vi "Annotating a Picture.vi"() -> ()   [LabVIEW 2023]
doc: "This example demonstrates how to add annotations, or additional images, to a starting image in a <b>2D Picture</b> indicator. The example keeps track of the parts of the image that have been annotated so that the annotations can also be removed if necessary. Finally, the example includes a button to save the modified image (including annotations) to a new image file."
uses:
  <vilib>/Utility/miscctls.llb/LVPoint32TypeDef.ctl
panel:
  in  "Save Image":bool
  in  "Stop":bool
  in  "Load Image":bool
  out "Image":picture
  # "Overview: Demonstrates how to add images as annotations to an existing image displayed in a 2D Picture indicator.\nInstructions: \n1. Run the VI.\n2. Click Load Image to load a JPG file into the picture indicator (this example loads the 'sample_board.jpg' image file).\n3. Right-click in the picture and select one of the Draw Annotation options. Observe the annotation that is added to the image.\n4. Right-click any annotation you have created and select Remove Annotation to see it be removed from the image.\n5. Click Save Image to save the image to a new JPG file. The new JPG file will contain the original image, along with any annotations that were created.\n6. Click Stop to stop the VI."
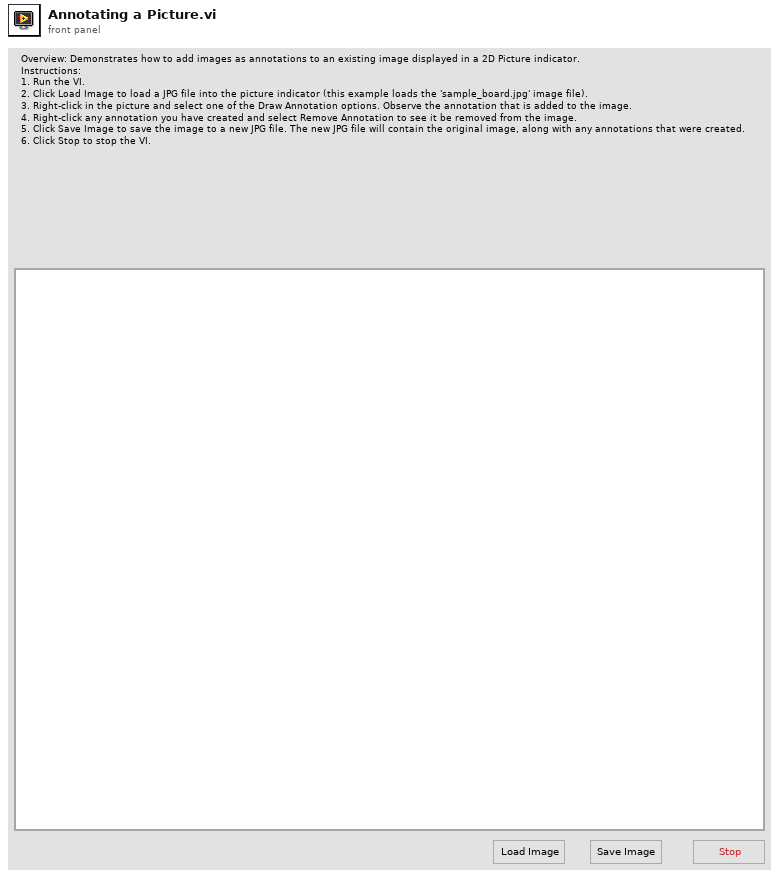
[diagram p1: front panel]
types:
  T1 = cluster{"left":i16, "top":i16, "right":i16, "bottom":i16}[]
  T2 = typedef "LVPoint32TypeDef.ctl" = cluster{"Horizontal":i32, "Vertical":i32}
  T3 = typedef "imagedata.ctl" = cluster{"image type":i32, "image depth":i32, "image":u8[], "mask":u8[], "colors":u32[], "Rectangle":cluster{"left":i16, "top":i16, "right":i16, "bottom":i16}}
  T4 = cluster{"left":i16, "top":i16, "right":i16, "bottom":i16}
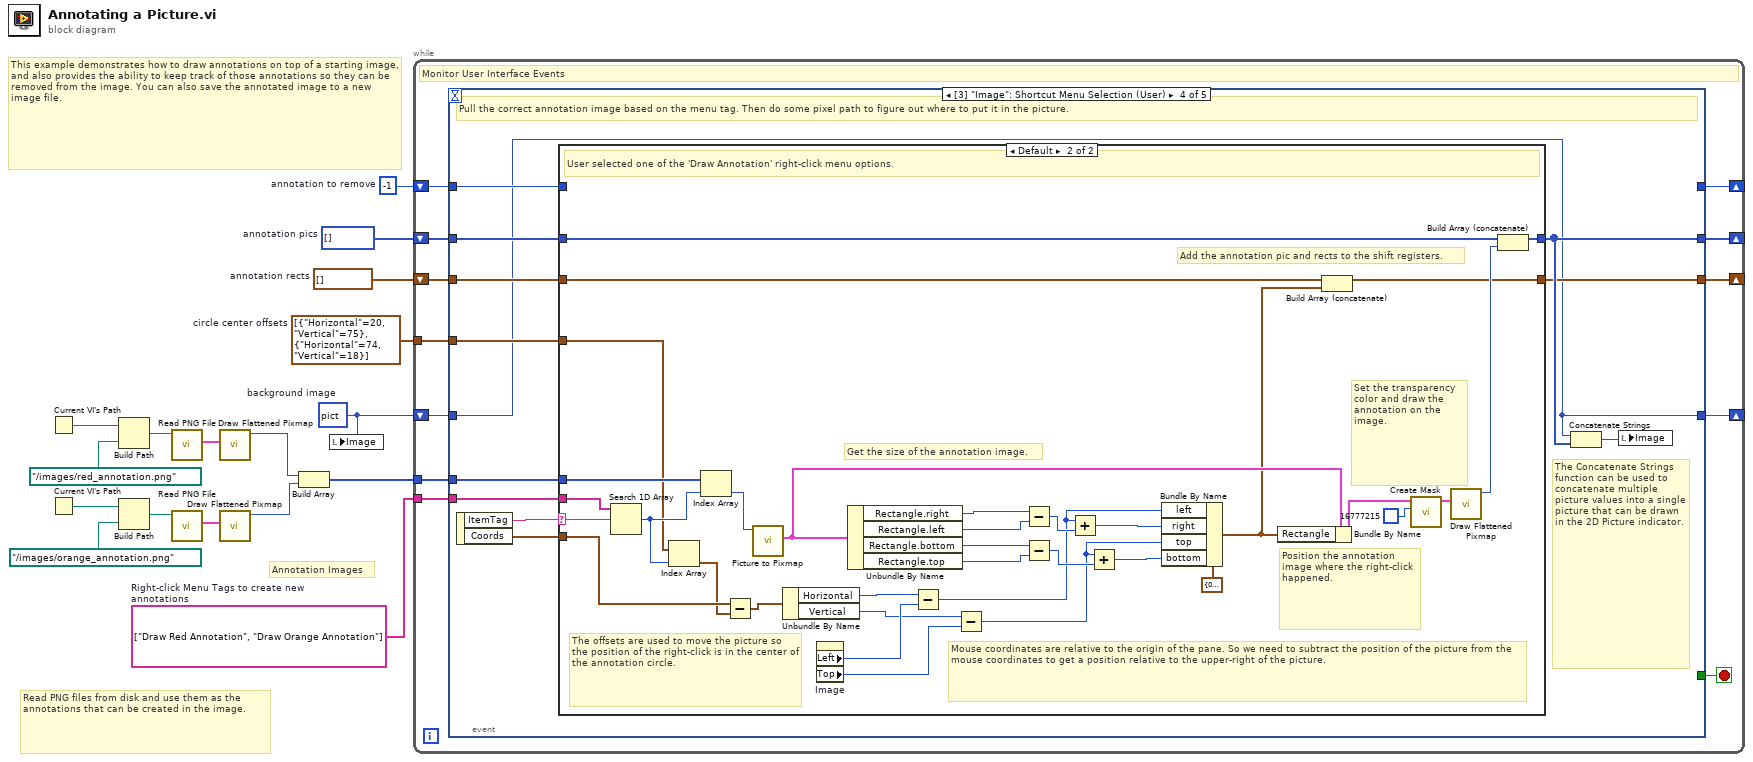
[diagram p0: block diagram]
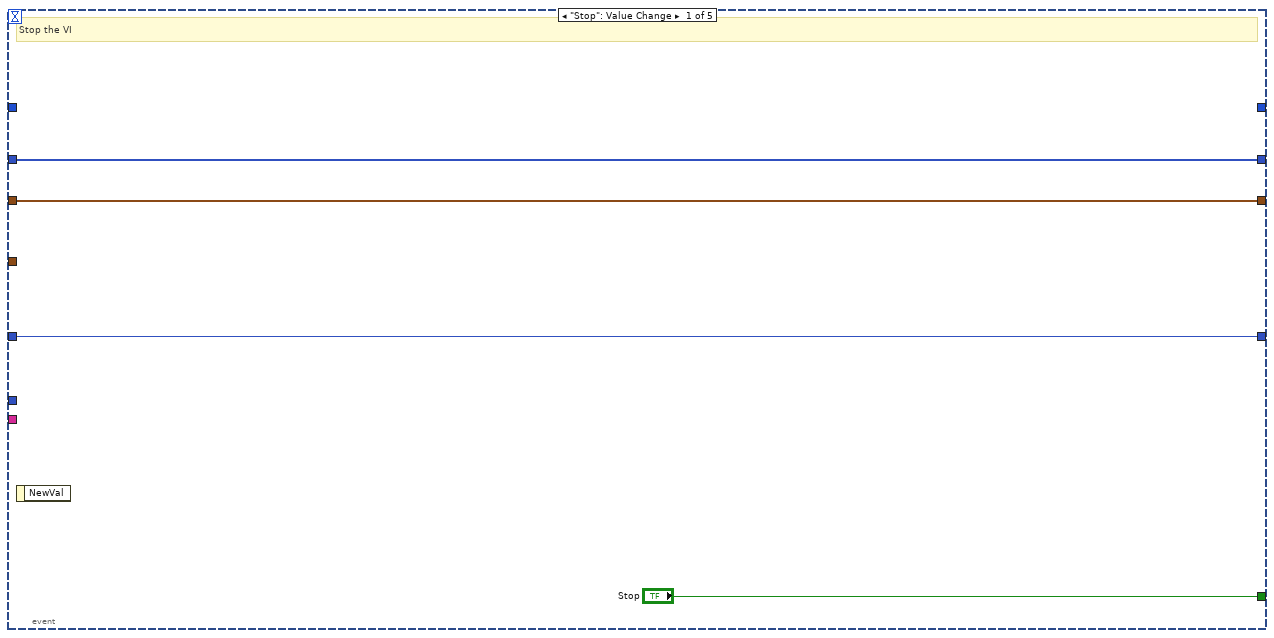
[diagram p2: hidden frame]
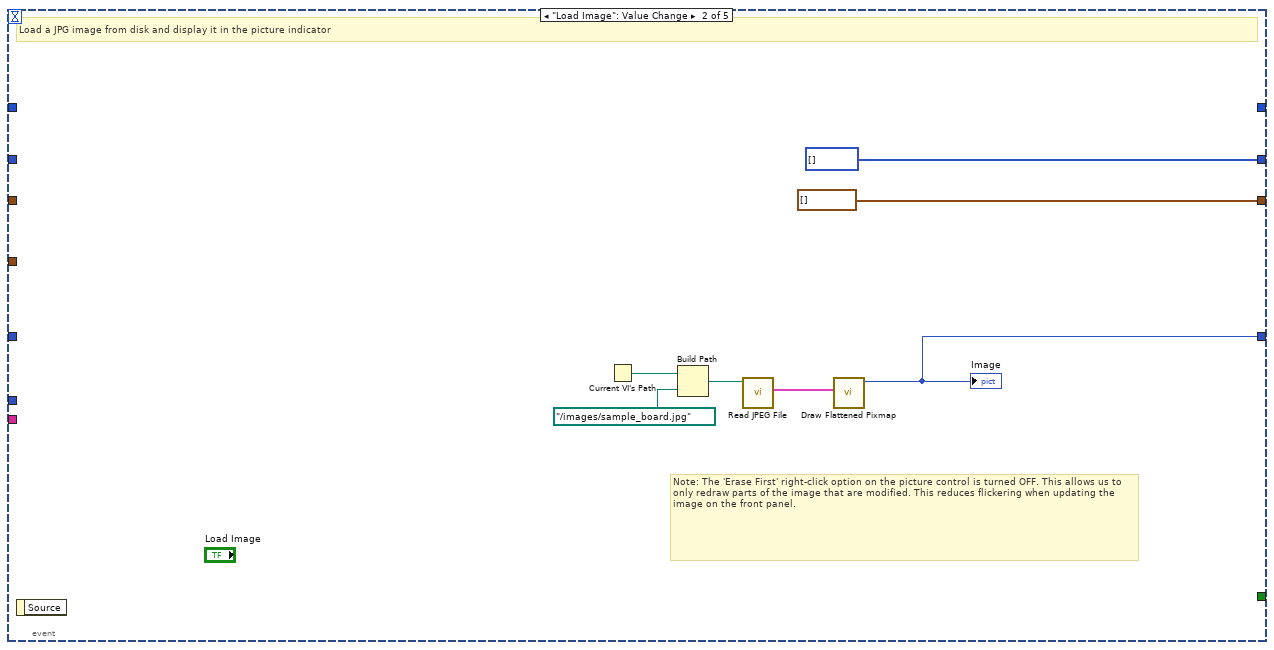
[diagram p3: hidden frame]
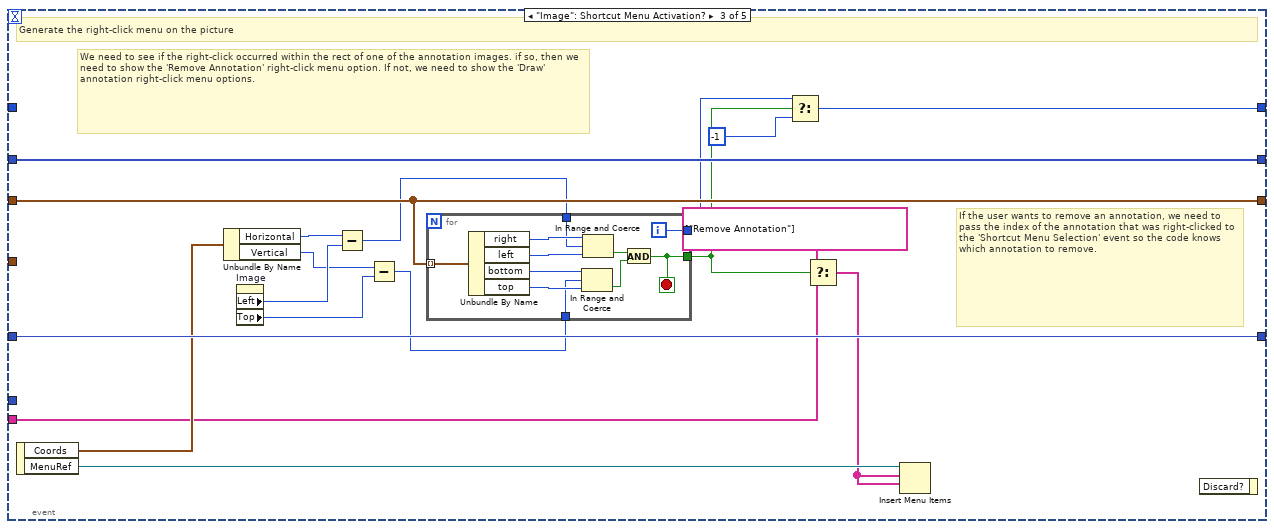
[diagram p4: hidden frame]
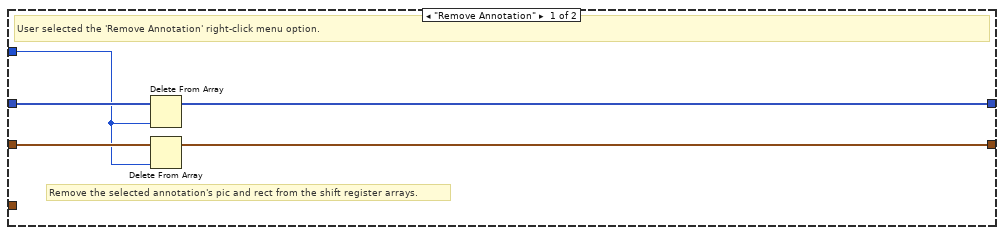
[diagram p5: hidden frame]
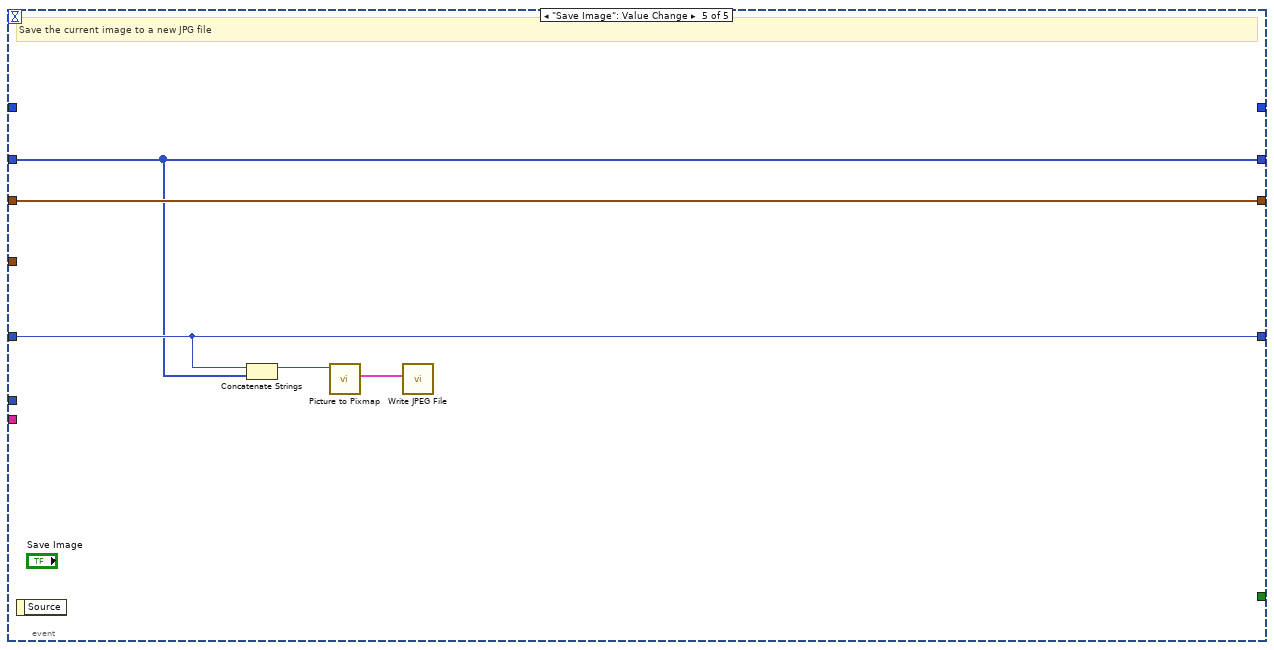
[diagram p6: hidden frame]
diagram:
  w9 = -1  # annotation to remove
  w10 = picture[] []  # annotation pics
  w11 = T1 []  # annotation rects
  w12 = T2[] [{"Horizontal"=20, "Vertical"=75}, {"Horizontal"=74, "Vertical"=18}]  # circle center offsets
  w15 = picture data[5B]  # background image
  w17 = string[] ["Draw Red Annotation", "Draw Orange Annotation"]  # Right-click Menu Tags to create new annotations
  # "This example demonstrates how to draw annotations on top of a starting image, and also provides the ability to keep track of those annotations so they can be removed from the image. You can also save the annotated image to a new image file."
  # "Annotation Images"
  # "Read PNG files from disk and use them as the annotations that can be created in the image."
  n1 = Current VI's Path() -> (path=w8:path)
  n2 = Current VI's Path() -> (path=w1:path)
  n3 = Build Path(base path=w8, name or relative path=path "../images/red_annotation.png") -> (appended path=w7:path)
  n4 = Build Path(base path=w1, name or relative path=path "../images/orange_annotation.png") -> (appended path=w2:path)
  n5 = call <vilib>:"Read PNG File.vi"("path to PNG file"=w7) -> ("image data"=w5:T3)  [unwired: 8 in, 2 out]
  n6 = call <vilib>:"Read PNG File.vi"("path to PNG file"=w2) -> ("image data"=w4:T3)  [unwired: 8 in, 2 out]
  n7 = call <vilib>:"Draw Flattened Pixmap.vi"("image data"=w5) -> ("new picture"=w14:picture)  [unwired: 8 in]
  n8 = call <vilib>:"Draw Flattened Pixmap.vi"("image data"=w4) -> ("new picture"=w13:picture)  [unwired: 8 in]
  n9 = Build Array(w14, w13) -> (w16:picture[])
  n10 = local write "Image"(w15) -> ()
  n11 = while {
    tunnel: w17 -> [w28]
    tunnel: w16 -> [w27]
    shift-right: [w25] -> _
    shift-left: w15 -> [w26]
    tunnel: w12 -> [w24]
    shift-right: [w22] -> _
    shift-left: w11 -> [w23]
    shift-right: [w21] -> _
    shift-left: w10 -> [w20]
    shift-right: [w18] -> _
    shift-left: w9 -> [w19]
    stop <- w29 stop-if-true
    # "Monitor User Interface Events"
    n12 = event shown="[3] \"Image\": Shortcut Menu Selection (User)" {
      selector: _ -> [_ _ _ _ _]
      dyn-events: _ -> [_ _ _ _ _]
      timeout: _ -> [_ _ _ _ _]
      tunnel: ["Stop" _ _ _ _] -> w29
      tunnel: w28 -> [_ _ w48 w80 _]
      tunnel: w27 -> [_ _ _ w79 _]
      tunnel: w26 -> [w32 _ w57 w70 w125]
      tunnel: [w32 w39 w57 w70 w125] -> w25
      tunnel: w24 -> [_ _ _ w76 _]
      tunnel: [w31 T1 [] ("annotation rects") w50 w72 w123] -> w22
      tunnel: w23 -> [w31 _ w50 w75 w123]
      tunnel: [w30 picture[] [] ("annotation pics") w56 w73 w121] -> w21
      tunnel: w20 -> [w30 _ w56 w74 w121]
      tunnel: w19 -> [_ _ _ w71 _]
      tunnel: [_ _ w42 _ _] -> w18
      event "Stop": Value Change {
        # "Stop the VI"
        n13 = event-data() -> ()  [unwired: 1 in, 1 out]
      }
      event "Load Image": Value Change {
        # "Note: The 'Erase First' right-click option on the picture control is turned OFF. This allows us to only redraw parts of the image that are modified. This reduces flickering when updating the image on the front panel."
        # "Load a JPG image from disk and display it in the picture indicator"
        n14 = event-data() -> ()  [unwired: 1 in, 1 out]
        n15 = Current VI's Path() -> (path=w36:path)
        n16 = Build Path(base path=w36, name or relative path=path "../images/sample_board.jpg") -> (appended path=w34:path)
        n17 = call <vilib>:"Read JPEG File.vi"("path to JPEG file"=w34) -> ("image data"=w40:T3)  [unwired: 8 in, 2 out]
        n18 = call <vilib>:"Draw Flattened Pixmap.vi"("image data"=w40) -> ("new picture"=w39:picture)  [unwired: 8 in]
        "Image" <- w39
      }
      event "Image": Shortcut Menu Activation? {
        # "If the user wants to remove an annotation, we need to pass the index of the annotation that was right-clicked to the 'Shortcut Menu Selection' event so the code knows which annotation to remove."
        # "We need to see if the right-click occurred within the rect of one of the annotation images. if so, then we need to show the 'Remove Annotation' right-click menu option. If not, we need to show the 'Draw' annotation right-click menu options."
        # "Generate the right-click menu on the picture"
        n19 = event-data() -> ("Coords"=w55:T2, "MenuRef"=w58:refnum<k9>)  [unwired: 1 in]
        n20 = Unbundle By Name(w55) -> ("Horizontal"=w54:i32, "Vertical"=w52:i32)
        n21 = property on="Image" class="Pict"() -> ("Left"=w53:i32, "Top"=w51:i32)  [unwired: 2 in, 2 out]
        n22 = Subtract(x=w54, y=w53) -> (x-y=w46:i32)
        n23 = Subtract(x=w52, y=w51) -> (x-y=w45:i32)
        n24 = for {
          tunnel: w50 -> [w69] mode=indexing
          tunnel: [w62] -> w44
          tunnel: w46 -> [w61]
          tunnel: w45 -> [w60]
          tunnel: [w59] -> w43
          i -> [w59]
          stop <- w62 stop-if-true
          n25 = Unbundle By Name(w69) -> ("right"=w68:i16, "left"=w67:i16, "bottom"=w66:i16, "top"=w65:i16)
          n26 = In Range and Coerce(upper limit=w66, x=w60, lower limit=w65) -> (In Range?=w63:bool)  [unwired: 1 out]
          n27 = In Range and Coerce(upper limit=w68, x=w61, lower limit=w67) -> (In Range?=w64:bool)  [unwired: 1 out]
          n28 = And(x=w64, y=w63) -> (x .and. y?=w62:bool)
        }
        n29 = Select(t=w43, s=w44, f=-1) -> (s? t:f=w42:i32)
        n30 = Select(t=string[] ["Remove Annotation"], s=w44, f=w48) -> (s? t:f=w47:string[])
        n31 = Insert Menu Items(7:w47, 8:w47, 9:w58) -> ()  [unwired: 3 in, 3 out]
        n32 = event-data() -> ()  [unwired: 2 in, 1 out]
      }
      event "Image": Shortcut Menu Selection (User) {
        # "The Concatenate Strings function can be used to concatenate multiple picture values into a single picture that can be drawn in the 2D Picture indicator."
        # "Pull the correct annotation image based on the menu tag. Then do some pixel path to figure out where to put it in the picture."
        n33 = event-data() -> ("ItemTag"=w81:string, "Coords"=w78:T2)  [unwired: 1 in]
        n34 = case shown="Default" w81 {
          selector: w81 -> [_ w120]
          tunnel: w80 -> [_ w119]
          tunnel: w79 -> [_ w118]
          tunnel: w78 -> [_ w113]
          tunnel: w76 -> [_ w93]
          tunnel: w75 -> [w84 w92]
          tunnel: w74 -> [w86 w90]
          tunnel: [w85 w89] -> w73
          tunnel: [w83 w88] -> w72
          tunnel: w71 -> [w82 _]
          frame "Remove Annotation" {
            # "Remove the selected annotation's pic and rect from the shift register arrays."
            # "User selected the 'Remove Annotation' right-click menu option."
            n35 = Delete From Array(array=w86, index=w82) -> (array with subset deleted=w85:picture[])  [unwired: 1 in, 1 out]
            n36 = Delete From Array(array=w84, index=w82) -> (array with subset deleted=w83:T1)  [unwired: 1 in, 1 out]
          }
          frame Default {
            # "Add the annotation pic and rects to the shift registers."
            # "The offsets are used to move the picture so the position of the right-click is in the center of the annotation circle."
            # "Set the transparency color and draw the annotation on the image."
            # "Position the annotation image where the right-click happened."
            # "Get the size of the annotation image."
            # "Mouse coordinates are relative to the origin of the pane. So we need to subtract the position of the picture from the mouse coordinates to get a position relative to the upper-right of the picture."
            # "User selected one of the 'Draw Annotation' right-click menu options."
            n37 = Search 1D Array(1D array=w119, element=w120) -> (index of element=w96:i32)  [unwired: 1 in]
            n38 = Index Array(array=w93, index=w96) -> (element=w94:T2)
            n39 = Index Array(array=w118, index=w96) -> (element=w115:picture)
            n40 = Subtract(x=w113, y=w94) -> (x-y=w95:T2)
            n41 = call <vilib>:"Picture to Pixmap.vi"("picture"=w115) -> ("image data"=w104:T3)  [unwired: 9 in, 1 out]
            n42 = Unbundle By Name(w95) -> ("Horizontal"=w101:i32, "Vertical"=w99:i32)
            n43 = property on="Image" class="Pict"() -> ("Left"=w102:i32, "Top"=w100:i32)  [unwired: 2 in, 2 out]
            n44 = Unbundle By Name(w104) -> ("Rectangle.right"=w112:i16, "Rectangle.left"=w111:i16, "Rectangle.bottom"=w108:i16, "Rectangle.top"=w107:i16)
            n45 = Subtract(x=w101, y=w102) -> (x-y=w98:i32)
            n46 = Subtract(x=w99, y=w100) -> (x-y=w97:i32)
            n47 = Subtract(x=w112, y=w111) -> (x-y=w110:i16)
            n48 = Subtract(x=w108, y=w107) -> (x-y=w105:i16)
            n49 = Add(x=w98, y=w110) -> (x+y=w109:i32)
            n50 = Add(x=w97, y=w105) -> (x+y=w106:i32)
            n51 = Bundle By Name(cluster=T4 {"left"=0, "top"=0, "right"=0, "bottom"=0} ("rect"), "left"=w98, "right"=w109, "top"=w97, "bottom"=w106) -> (w87:T4)
            n52 = Bundle By Name(cluster=w104, "Rectangle"=w87) -> (w103:T3)
            n53 = Build Array (concatenate)(w92, w87) -> (w88:T1)
            n54 = call <vilib>:"Create Mask.vi"("Mask Color (Black)"=u32 16777215, "image data"=w103) -> ("image data"=w117:T3)  [unwired: 9 in]
            n55 = call <vilib>:"Draw Flattened Pixmap.vi"("image data"=w117) -> ("new picture"=w91:picture)  [unwired: 8 in]
            n56 = Build Array (concatenate)(w90, w91) -> (w89:picture[])
          }
        }
        n57 = Concatenate Strings(w70, w73) -> (w77:picture)
        n58 = local write "Image"(w77) -> ()
      }
      event "Save Image": Value Change {
        # "Save the current image to a new JPG file"
        n59 = event-data() -> ()  [unwired: 1 in, 1 out]
        n60 = Concatenate Strings(w125, w121) -> (w122:picture)
        n61 = call <vilib>:"Picture to Pixmap.vi"("picture"=w122) -> ("image data"=w124:T3)  [unwired: 9 in, 1 out]
        n62 = call <vilib>:"Write JPEG File.vi"("image data"=w124) -> ()  [unwired: 9 in, 2 out]
      }
    }
  }
